vi "frontEnd.vi"(8 "error in (no error)":errorcluster, 10 "HWControllerEvents":refnum<class "HWControllerEvents.lvclass">, 11 "CameraControlViewer in":refnum<class "CameraControlViewer.lvclass">) -> (0 "error out":errorcluster, 3 "CameraControlViewer out":refnum<class "CameraControlViewer.lvclass">)   [LabVIEW 2011, in "Views.lvlib" / "Camera.lvlib" / "CameraControlViewer.lvclass"]
uses:
  CameraControlViewer.lvclass
  Hal/HWController/HWControllerEvents/HWControllerEvents.lvclass
  CameraControlViewer.lvclass/CameraControlViewer.ctl
  Tools/Filing/FileNeologist/FileNeologist.lvclass
  Tools/Filing.lvlib
panel:
  in  "Camera":enum16{"Pixis", "ProEM", "PixelFly"}(ring)
  in  "upload":bool
  in  "stop":bool
  in  "start":bool
  # "-1 is video mode"
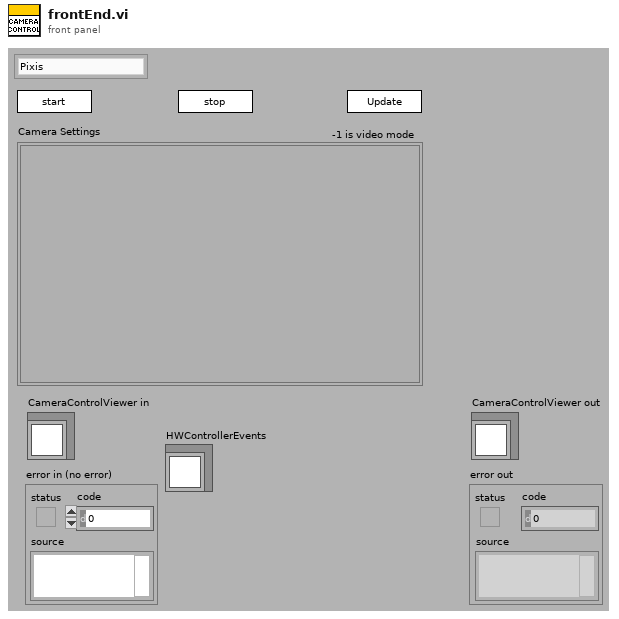
[diagram p1: front panel]
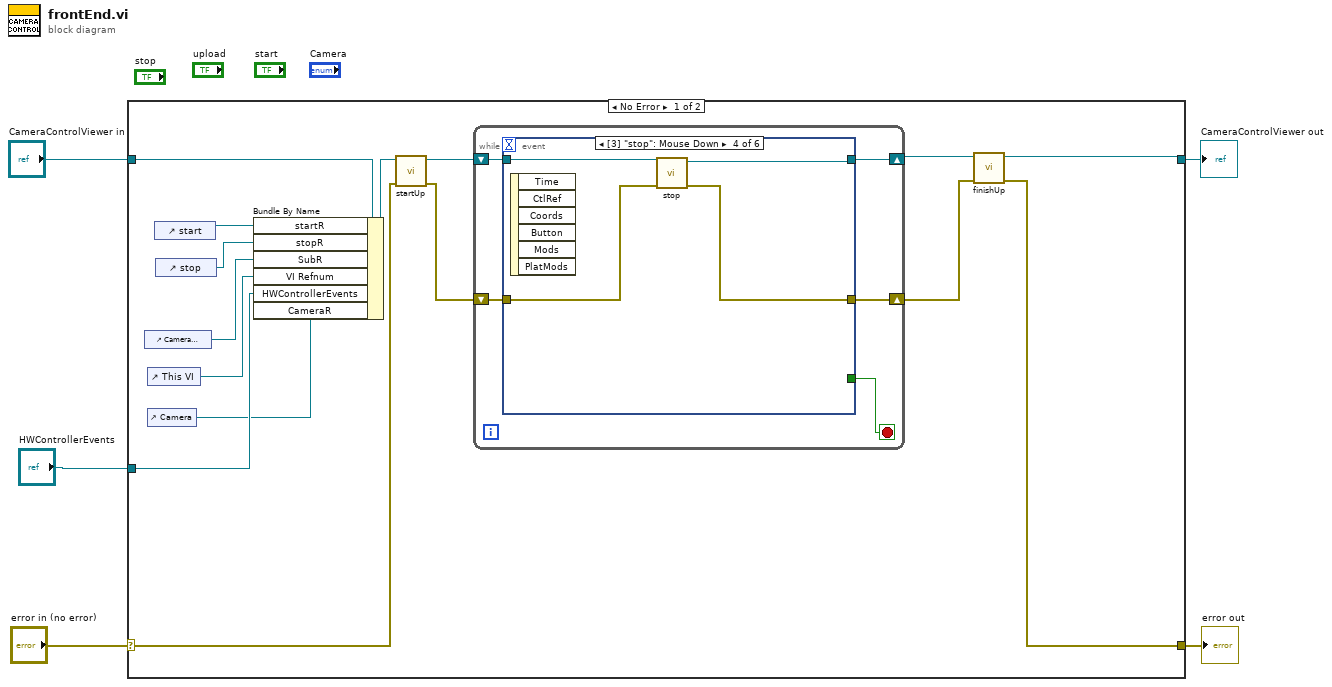
[diagram p0: block diagram]
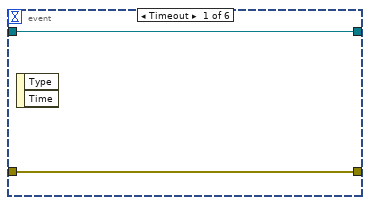
[diagram p2: hidden frame]
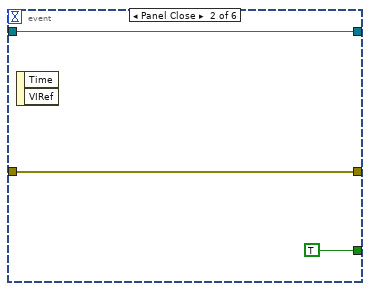
[diagram p3: hidden frame]
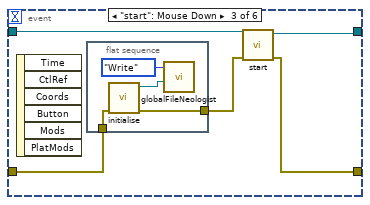
[diagram p4: hidden frame]
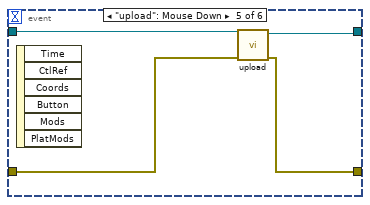
[diagram p5: hidden frame]
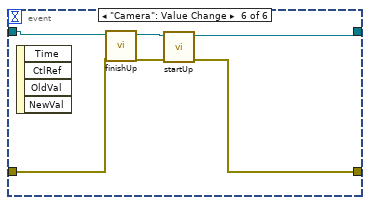
[diagram p6: hidden frame]
diagram:
  n1 = case shown="No Error" "error in (no error)" {
    selector: "error in (no error)" -> [w14 w55]
    tunnel: [w9 w55] -> w4
    tunnel: [w11 w54] -> w2
    tunnel: "CameraControlViewer in" -> [w17 w54]
    tunnel: "HWControllerEvents" -> [w7 _]
    frame No Error {
      n2 = control-ref of="Camera Settings"() -> (w18:refnum<vi>)
      n3 = control-ref of="This VI"() -> (w8:refnum<vi>)
      n4 = control-ref of="Camera"() -> (w6:refnum<vi>)
      n5 = control-ref of="start"() -> (w20:refnum<vi>)
      n6 = control-ref of="stop"() -> (w19:refnum<vi>)
      n7 = Bundle By Name(cluster=w17, "startR"=w20, "stopR"=w19, "SubR"=w18, "VI Refnum"=w8, "HWControllerEvents"=w7, "CameraR"=w6) -> (w16:refnum<class "CameraControlViewer.lvclass">)
      n8 = call "startUp.vi"("error in (no error)"=w14, "CameraControlViewer in"=w16) -> ("error out"=w13:errorcluster, "CameraControlViewer out"=w15:refnum<class "CameraControlViewer.lvclass">)  [unwired: 8 in]
      n9 = while {
        shift-right: [w24] -> w12
        shift-left: w15 -> [w25]
        shift-right: [w22] -> w10
        shift-left: w13 -> [w23]
        stop <- w21 stop-if-true
        n10 = event shown="[3] \"stop\": Mouse Down" {
          selector: _ -> [_ _ _ _ _ _]
          dyn-events: _ -> [_ _ _ _ _ _]
          timeout: _ -> [_ _ _ _ _ _]
          tunnel: w25 -> [w27 w30 w35 w43 w47 w53]
          tunnel: [w27 w30 w34 w42 w46 w49] -> w24
          tunnel: w23 -> [w26 w29 w32 w41 w45 w52]
          tunnel: [w26 w29 w33 w40 w44 w48] -> w22
          tunnel: [_ TRUE _ _ _ _] -> w21
          event Timeout {
            n11 = event-data() -> ()  [unwired: 1 in, 2 out]
          }
          event Panel Close {
            n12 = event-data() -> ()  [unwired: 1 in, 2 out]
          }
          event "start": Mouse Down {
            n13 = event-data() -> ()  [unwired: 1 in, 6 out]
            n14 = flat-sequence {
              tunnel: w32 -> [w37]
              tunnel: [w36] -> w31
              frame #0 {
                n15 = call "initialise.vi"("error in (no error)"=w37) -> ("error out"=w36:errorcluster, "FileNeologist out"=w38:refnum<class "FileNeologist.lvclass">)  [unwired: 9 in]
                n16 = call "globalFileNeologist.vi"("FileNeologist in"=w38, "Action"=enum16{"Write", "Read"}."Write") -> ()  [unwired: 9 in, 1 out]
              }
            }
            n17 = call "start.vi"("error in (no error)"=w31, "CameraControlViewer in"=w35) -> ("error out"=w33:errorcluster, "CameraControlViewer out"=w34:refnum<class "CameraControlViewer.lvclass">)  [unwired: 8 in]
          }
          event "stop": Mouse Down {
            n18 = event-data() -> ()  [unwired: 1 in, 6 out]
            n19 = call "stop.vi"("error in (no error)"=w41, "CameraControlViewer in"=w43) -> ("error out"=w40:errorcluster, "CameraControlViewer out"=w42:refnum<class "CameraControlViewer.lvclass">)  [unwired: 8 in]
          }
          event "upload": Mouse Down {
            n20 = event-data() -> ()  [unwired: 1 in, 6 out]
            n21 = call "upload.vi"("error in (no error)"=w45, "CameraControlViewer in"=w47) -> ("error out"=w44:errorcluster, "CameraControlViewer out"=w46:refnum<class "CameraControlViewer.lvclass">)  [unwired: 8 in]
          }
          event "Camera": Value Change {
            n22 = event-data() -> ()  [unwired: 1 in, 4 out]
            n23 = call "finishUp.vi"("error in (no error)"=w52, "CameraControlViewer in"=w53) -> ("error out"=w50:errorcluster, "CameraControlViewer out"=w51:refnum<class "CameraControlViewer.lvclass">)  [unwired: 8 in]
            n24 = call "startUp.vi"("error in (no error)"=w50, "CameraControlViewer in"=w51) -> ("error out"=w48:errorcluster, "CameraControlViewer out"=w49:refnum<class "CameraControlViewer.lvclass">)  [unwired: 8 in]
          }
        }
      }
      n25 = call "finishUp.vi"("error in (no error)"=w10, "CameraControlViewer in"=w12) -> ("error out"=w9:errorcluster, "CameraControlViewer out"=w11:refnum<class "CameraControlViewer.lvclass">)  [unwired: 8 in]
    }
    frame Error {
    }
  }
  "error out" <- w4
  "CameraControlViewer out" <- w2
